vi "SaveDataSet.vi"(6 "AssetNodeMap":variant, 7 "do not write to database":bool, 8 "error in (no error)":errorcluster, 9 "Waveform":waveform(sgl), 10 "DataSetRegistry":T1, 11 "event in":T3) -> (0 "error out":errorcluster, 3 "event out":T3)   [LabVIEW 2017, in "McsaDataEventCreator.lvlib"]
uses:
  <vilib>/addons/InsightCM/Devices/Shared/Mcsa/McsaDataEventCreator/McsaDataEventCreator.lvlib
  <vilib>/addons/InsightCM/Devices/Shared/Common/DataEvent/controls/Event.ctl
  <vilib>/addons/InsightCM/MessageBus/Base/controls/DataEvent.ctl
  <vilib>/addons/InsightCM/MessageBus/Base/controls/KeyValuePair.ctl
  <vilib>/addons/InsightCM/Devices/Shared/Common/DataEvent/controls/DataSet.ctl
  <vilib>/addons/InsightCM/MessageBus/Base/controls/DataSetMetadata.ctl
  <vilib>/addons/InsightCM/MessageBus/Base/controls/TrendPoint.ctl
  <vilib>/addons/InsightCM/MessageBus/Base/controls/TrendAlarmUpdate.ctl
  <vilib>/addons/InsightCM/MessageBus/Base/controls/TrendAlarmTransition.ctl
  <vilib>/addons/InsightCM/Devices/Shared/Mcsa/McsaDataEventCreator/controls/Registry_DataSet.ctl
  <vilib>/addons/InsightCM/Devices/Shared/Mcsa/McsaDataEventCreator/controls/DataSetType.ctl
  <vilib>/addons/InsightCM/Devices/Shared/Common/DataEventCreator/DataEventCreator.lvlib
  <vilib>/addons/InsightCM/Devices/Shared/Common/DataEvent/DataEvent.lvlib
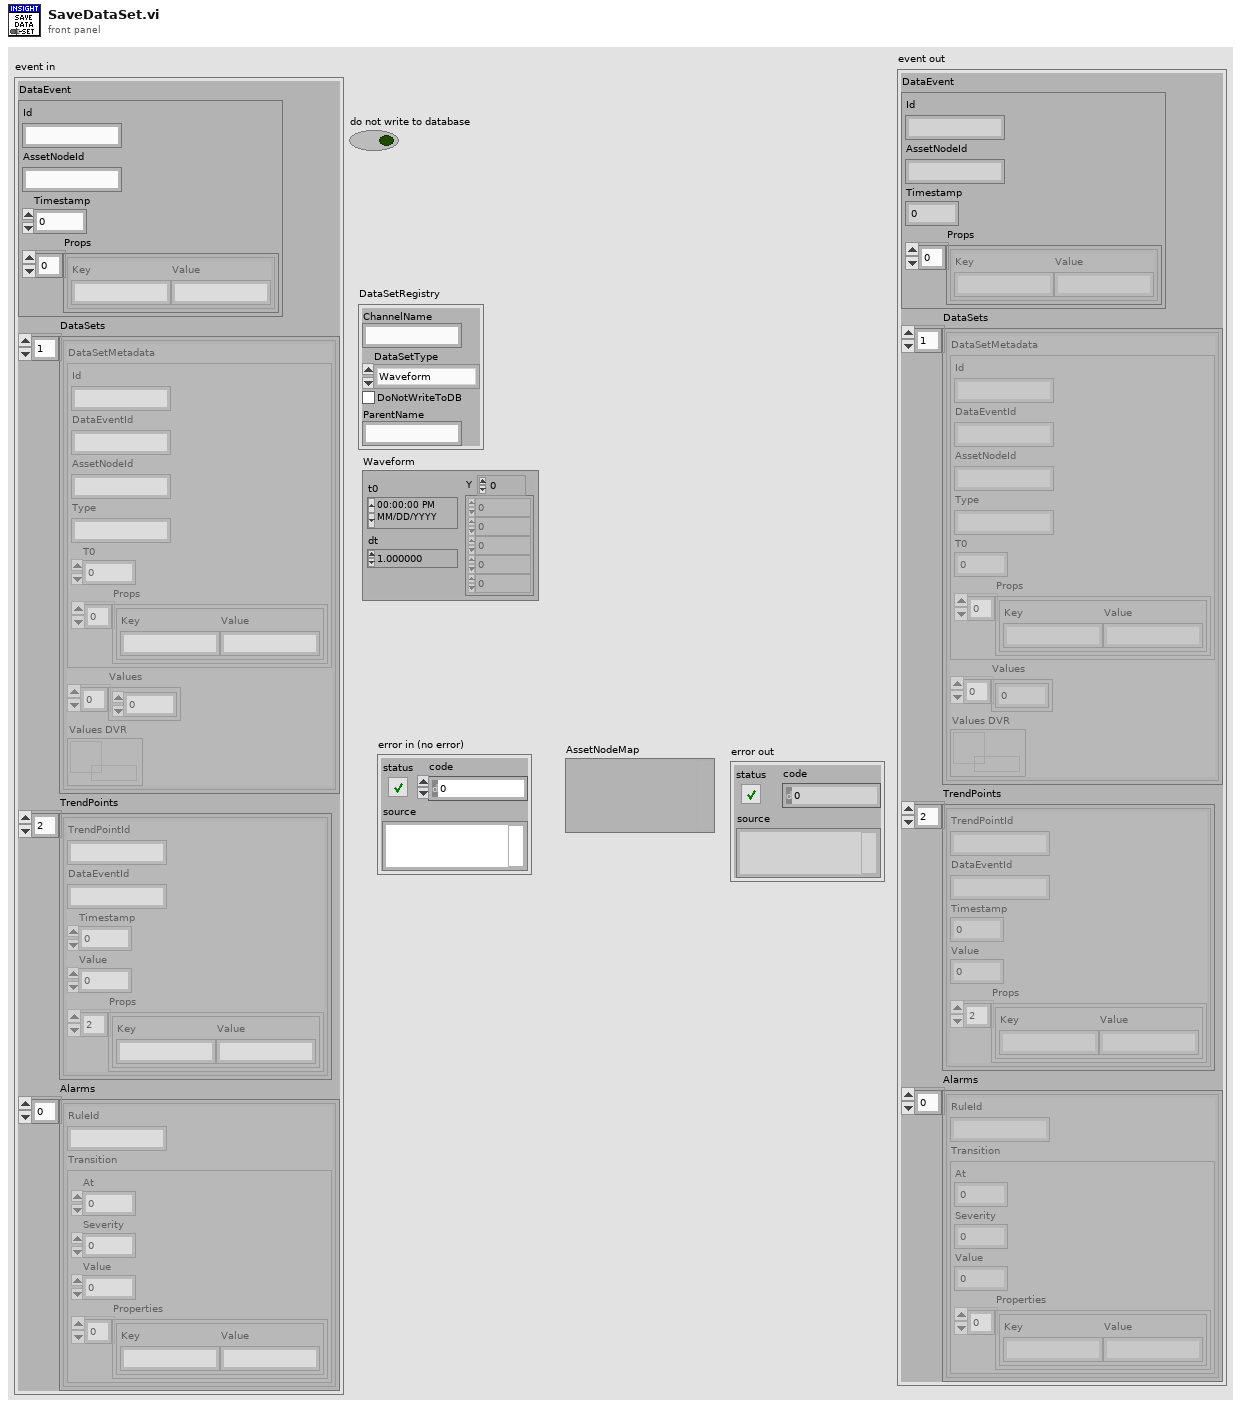
[diagram p1: front panel]
types:
  T1 = typedef "McsaDataEventCreator.lvlib/Registry_DataSet.ctl" = cluster{"ChannelName":string, "DataSetType":T2, "DoNotWriteToDB":bool, "ParentName":string}
  T2 = typedef "McsaDataEventCreator.lvlib/DataSetType.ctl" = enum16{"Waveform", "MCSAFFT", "TorqueWFM"}
  T3 = typedef "DataEvent.lvlib/Event.ctl" = cluster{"DataEvent":T4, "DataSets":T6[], "TrendPoints":T8[], "Alarms":T9[]}
  T4 = typedef "DataEvent.ctl" = cluster{"Id":string, "AssetNodeId":string, "Timestamp":i64, "Props":T5[]}
  T5 = typedef "KeyValuePair.ctl" = cluster{"Key":string, "Value":string}
  T6 = typedef "DataEvent.lvlib/DataSet.ctl" = cluster{"DataSetMetadata":T7, "Values":sgl[], "Values DVR":refnum<data-value>}
  T7 = typedef "DataSetMetadata.ctl" = cluster{"Id":string, "DataEventId":string, "AssetNodeId":string, "Type":string, "T0":i64, "Props":T5[]}
  T8 = typedef "TrendPoint.ctl" = cluster{"TrendPointId":string, "DataEventId":string, "Timestamp":i64, "Value":dbl, "Props":T5[]}
  T9 = typedef "TrendAlarmUpdate.ctl" = cluster{"RuleId":string, "Transition":T10}
  T10 = typedef "TrendAlarmTransition.ctl" = cluster{"At":i64, "Severity":i32, "Value":dbl, "Properties":T5[]}
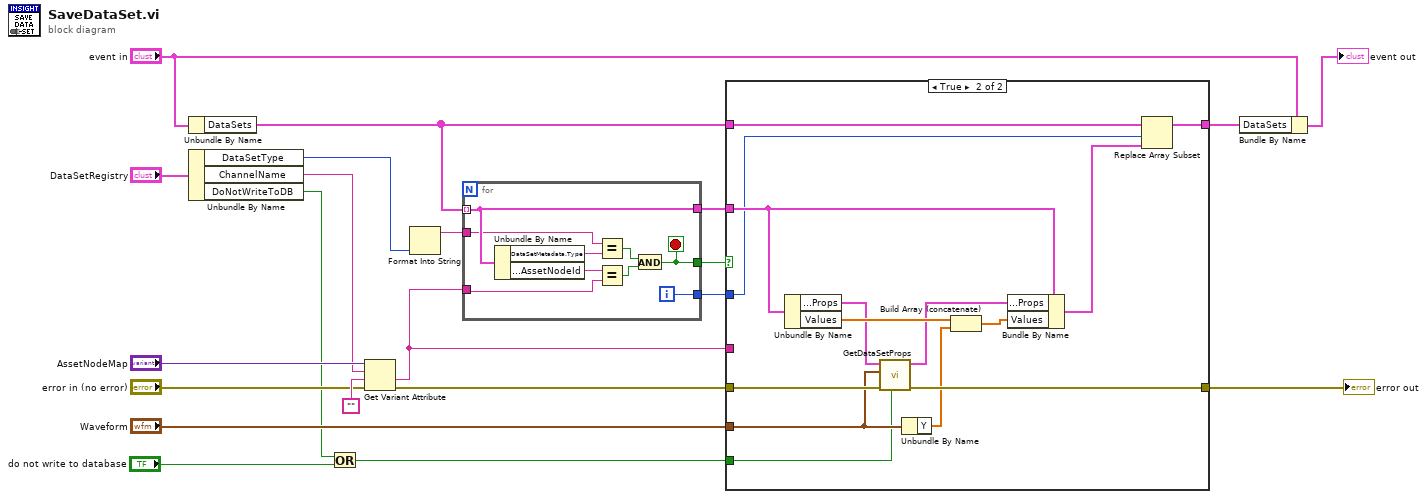
[diagram p0: block diagram]
diagram:
  n1 = Unbundle By Name("event in") -> ("DataSets"=w15:T6[])
  n2 = Unbundle By Name("DataSetRegistry") -> ("DataSetType"=w7:T2, "ChannelName"=w9:string, "DoNotWriteToDB"=w2:bool)
  n3 = Or(x=w2, y="do not write to database") -> (x .or. y?=w1:bool)
  n4 = Get Variant Attribute(Variant="AssetNodeMap", name=w9, default value (empty Variant)="", error in="error in (no error)") -> (value=w17:string, error out=w5:errorcluster)  [unwired: 2 out]
  n5 = Format Into String(w7) -> (resulting string=w6:string)  [unwired: 3 in, 1 out]
  n6 = for {
    tunnel: w15 -> [w28] mode=indexing
    tunnel: w17 -> [w29]
    tunnel: [w24] -> w18
    tunnel: [w28] -> w12
    tunnel: [w27] -> w11
    tunnel: w6 -> [w22]
    i -> [w27]
    stop <- w24 stop-if-true
    n7 = Unbundle By Name(w28) -> ("DataSetMetadata.Type"=w23:string, "DataSetMetadata.AssetNodeId"=w30:string)
    n8 = Equal?(x=w22, y=w23) -> (x = y?=w26:bool)
    n9 = Equal?(x=w30, y=w29) -> (x = y?=w25:bool)
    n10 = And(x=w26, y=w25) -> (x .and. y?=w24:bool)
  }
  n11 = case shown="True" w18 {
    tunnel: w5 -> [w31 w39]
    tunnel: w17 -> [_ _]
    tunnel: w15 -> [w32 w43]
    tunnel: [w32 w42] -> w14
    tunnel: w12 -> [_ w45]
    tunnel: w11 -> [_ w41]
    tunnel: [w31 w38] -> w8
    tunnel: "Waveform" -> [_ w35]
    tunnel: w1 -> [_ w33]
    frame False {
    }
    frame True {
      n12 = Unbundle By Name(w45) -> ("DataSetMetadata.Props"=w34:T5[], "Values"=w46:sgl[])
      n13 = call <vilib>:"GetDataSetProps.vi"("do not write to database"=w33, "error in (no error)"=w39, "waveform"=w35, "dataset props in"=w34) -> ("error out"=w38:errorcluster, "dataset props out"=w37:T5[])  [unwired: 6 in]
      n14 = Unbundle By Name(w35) -> ("Y"=w36:sgl[])
      n15 = Build Array (concatenate)(w46, w36) -> (w44:sgl[])
      n16 = Bundle By Name(cluster=w45, "DataSetMetadata.Props"=w37, "Values"=w44) -> (w40:T6)
      n17 = Replace Array Subset(array=w43, new element=w40, index=w41) -> (w42:T6[])
    }
  }
  "error out" <- w8
  n18 = Bundle By Name(cluster="event in", "DataSets"=w14) -> (→"event out":T3)
